vi "tkrsa6100 Write-Read wError Query.vi"(0 "VISA Resource Name":refnum<visa-resource-name>, 1 "Max Read Byte\nCount (1000)":i32=1000 min=1000 max=1000000 step=1000, 5 "Error Query(YES)":enum16{"NO", "YES"}(ring)=enum."YES", 7 "Command (Empty String)":string, 9 "Response String \nFormat(ASCII)":enum16{"ASCII", "BINARY"}(ring), 11 "error in (no error)":errorcluster, 12 "Timeout(S) (10)":i32=10) -> (4 "dup VISA Resource Name":refnum<visa-resource-name>, 6 "Response":string, 8 "Byte Count Xfrd":i32, 15 "error out":errorcluster {"code" format="%#.0f"})   [LabVIEW 2020, in "Library Instrument & Equipement.lvlib" / "Library Spectrum Analyser.lvlib"]
doc: "Prerequisites for use: \nThis VI is valid in all measurements.\n\nThis VI controls the following functions.\nWrites GPIB commands\nReads GPIB query responses\nAdds an error query to writes/reads depending on user input. This is done to avoid a timeout condition that will occur if a query is sent in an invalid measurement.\n\nerror in (no error) is checked for any pending errors.\n\nIf error in status is ERROR:\n\nerror in (no error) and VISA Resource Name are passed straight through to error out and dup VISA Resource Name and returned to the calling function. No commands are processed.\n\nIf error in status is NO ERROR:\n\nPass the following parameters.\n\nCommand (Empty String)\nCommand or query to send.\n\nResponse String Format (ASCII)\nPass ASCII for queries that return ascii text strings.\nPass BINARY for queries that return binary blocks.\n\nMax Read Byte Count (1000)\nThe default value (1000) is adequate for most queries except for binary blocks which will require a higher count.\n\nTimeout (S) (30)\nThis defaults to 30 seconds which should be adequate for most applications. If not pass the desired timeout in seconds.\n\nError Query (YES)\nThis defaults to YES which will append an error query to the command/query string sent. If no error query is to be sent, pass NO to this input.\n\nOne command/query is executed per VI call\n\nInformation returned by the VI is:\n\ndup VISA Resource Name\nError Out\n\nResponse. \nString returned by the current query\n\nByte Count Xfered. \n# of bytes returned by the current query\n\nThe VI functions as follows:\n\nThe first sequence frame simply clears Response with an empty string.\n\nThe desired GPIB timeout is set via the user input to the property node.\n\nThe VISA Write function receives the command/query passed by the user and depending on the setting of Error Query (YES) appends <:syst:err?> or an empty string to Command (Empty String).\n\nThe VISA Read function in the following case structure is executed either if Error Query (YES) is set to YES or if the current string in Command (Empty String) contains a \"?\" (instrument query). The maximum byte count is to be read is set by the value passed to Max Read Byte Count (1000). The default value is sufficient for most ASCII transfers but a larger value is necessary for binary block transfers. The actual byte count read is returned in indicator Byte Count Xfrd.\n\nThe final case structure executes as follows:\n\nIf Error Query (YES) is set to YES\nThe instrument query response and Error Out are passed to tkrsa6100 Error Parser.vi for further processing. tkrsa6100 Error Parser.vi returns the instrument query response and updated cluster Error Out.\n\nIf Error Query (YES) is set to NO and Response String Format (ASCII) is set to BINARY\nThe instrument response and Error Out are passed straight through to string indicator Response and cluster Error Out.\n\nIf Error Query (YES) is set to NO and Response String Format (ASCII) is set to ASCII\nthe instrument response is passed through tkrsa6100 Quote Stripper.vi which simply removes any quotes around responses. Some instrument responses are quoted, some are not. For consistency all instrument responses returned to the user are unquoted. If no quotes are present in the instrument response the VI outputs the same string as was input to it.\n\nOn completion dup VISA Resource Name, Error Out, Response, and Byte Count Xfrd are returned to the calling function."
uses:
  Library Spectrum Analyser.lvlib
panel:
  # "RSA6100 Write/Read w/Error Query Driver"
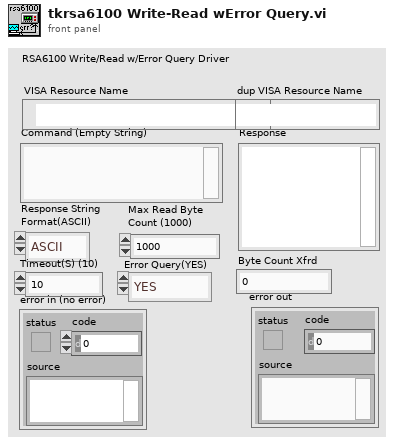
[diagram p1: front panel]
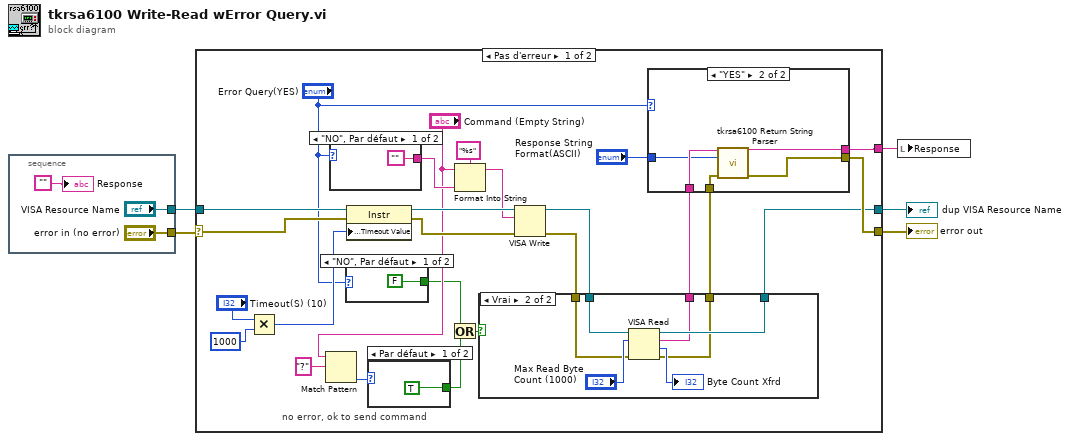
[diagram p0: block diagram]
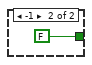
[diagram p2: hidden frame]
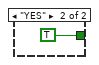
[diagram p3: hidden frame]
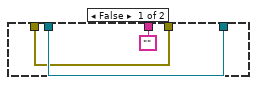
[diagram p4: hidden frame]
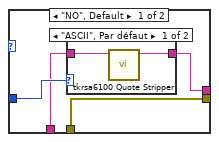
[diagram p5: hidden frame]
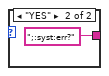
[diagram p7: hidden frame]
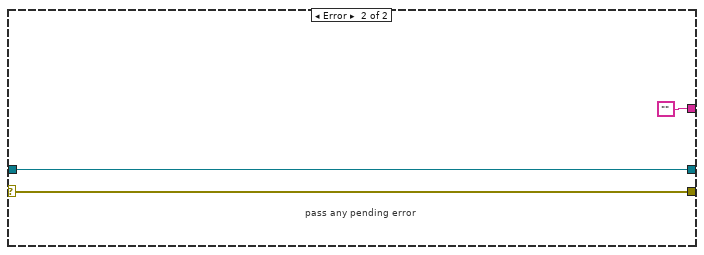
[diagram p8: hidden frame]
diagram:
  n1 = stacked-sequence {
    tunnel: ["VISA Resource Name"] -> w5
    tunnel: ["error in (no error)"] -> w2
    frame #0 {
      "Response" <- ""
    }
  }
  n2 = case shown="Pas d'erreur" w2 {
    selector: w2 -> [w30 w63]
    tunnel: w5 -> [w31 w64]
    tunnel: [w20 w64] -> w4
    tunnel: [w23 w63] -> w3
    tunnel: [w10 ""] -> w1
    frame No Error {
      # "no error, ok to send command"
      n3 = Multiply(x="Timeout(S) (10)", y=u32 1000) -> (x*y=w27:u32)
      n4 = Match Pattern(string="Command (Empty String)", regular expression="?" ("input 1")) -> (offset past match=w16:i32)  [unwired: 4 out]
      n5 = case shown="\"NO\", Par défaut" "Error Query(YES)" {
        tunnel: ["" ";:syst:err?" ("input 1")] -> w25
        frame "NO", Default {
        }
        frame "YES" {
        }
      }
      n6 = case shown="\"NO\", Par défaut" "Error Query(YES)" {
        tunnel: [FALSE TRUE] -> w14
        frame "NO", Default {
        }
        frame "YES" {
        }
      }
      n7 = property on="Property Node" class="Instr"(reference=w31, error in=w30, "General Settings:Timeout Value"=w27) -> (reference out=w33:refnum<visa-resource-name>, error out=w32:errorcluster)
      n8 = case shown="Par défaut" w16 {
        tunnel: [TRUE FALSE] -> w15
        frame Default {
        }
        frame -1 {
        }
      }
      n9 = Or(x=w14, y=w15) -> (x .or. y?=w19:bool)
      n10 = Format Into String(format string="%s", initial string="Command (Empty String)", w25) -> (resulting string=w24:string)  [unwired: 1 in, 1 out]
      n11 = VISA Write(VISA resource name=w33, write buffer=w24, error in (no error)=w32) -> (VISA resource name out=w22:refnum<visa-resource-name>, error out=w21:errorcluster)  [unwired: 1 out]
      n12 = case shown="Vrai" w19 {
        tunnel: w22 -> [w40 w45]
        tunnel: w21 -> [w38 w44]
        tunnel: ["" w42] -> w11
        tunnel: [w40 w43] -> w20
        tunnel: [w38 w41] -> w13
        frame False {
        }
        frame True {
          n13 = VISA Read(VISA resource name=w45, byte count="Max Read Byte\nCount (1000)", error in (no error)=w44) -> (VISA resource name out=w43:refnum<visa-resource-name>, read buffer=w42:string, return count=→"Byte Count Xfrd":u32, error out=w41:errorcluster)
        }
      }
      n14 = case shown="\"YES\"" "Error Query(YES)" {
        tunnel: [w48 w56] -> w10
        tunnel: [w51 w55] -> w23
        tunnel: w11 -> [w49 w59]
        tunnel: w13 -> [w51 w58]
        tunnel: "Response String \nFormat(ASCII)" -> [w50 w57]
        frame "NO", Default {
          n15 = case shown="\"ASCII\", Par défaut" w50 {
            tunnel: w49 -> [w53 w54]
            tunnel: [w52 w54] -> w48
            frame "ASCII", Default {
              n16 = call "tkrsa6100 Quote Stripper.vi"("Input String"=w53) -> ("Output String"=w52:string)  [unwired: 10 out]
            }
            frame "BINARY" {
            }
          }
        }
        frame "YES" {
          n17 = call "tkrsa6100 Return String Parser.vi"("Read Buffer"=w59, "Response String \nFormat(ASCII)"=w57, "error in (no error)"=w58) -> ("Inst Query Response"=w56:string, "error out"=w55:errorcluster)  [unwired: 11 out]
        }
      }
    }
    frame Error {
      # "pass any pending error"
    }
  }
  "error out" <- w3
  "dup VISA Resource Name" <- w4
  n18 = local write "Response"(w1) -> ()
